vi "c_ctre_phoenix6_free_memory.vi"(0 "Numeric 3":u32) -> (20 "Numeric":i32, 21 "Numeric 2":u32)   [LabVIEW 2023]
uses:
  <vilib>/Rock Robotics/WPI/ThirdParty/Phoenix-LabVIEW/Controls/DriverLib.ctl
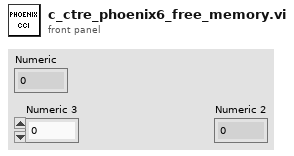
[diagram p1: front panel]
types:
  T1 = typedef "DriverLib.ctl" = path
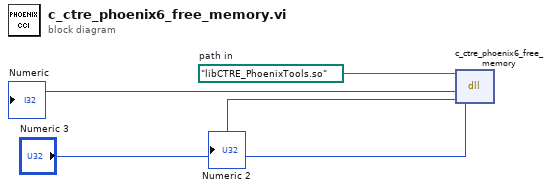
[diagram p0: block diagram]
diagram:
  w4 = T1 path "libCTRE_PhoenixTools.so"  # path in
  n1 = dll-call lib="?" fn="c_ctre_phoenix6_free_memory"(path in=w4, "Numeric 3") -> (→"Numeric":i32, →"Numeric 2":u64)  [unwired: 2 in, 2 out]
